vi "Init with SQL Record.vi"(8 "error in (no error)":errorcluster, 10 "MySQL Record":variant[](array[variant]), 11 "Banking Transaction in":refnum<class "Banking Transaction.lvclass">) -> (0 "error out":errorcluster, 3 "Banking Transaction out":refnum<class "Banking Transaction.lvclass">)   [LabVIEW 2018, in "Banking Transaction.lvclass"]
uses:
  Banking Transaction.lvclass
  Transaction/Transaction.lvclass
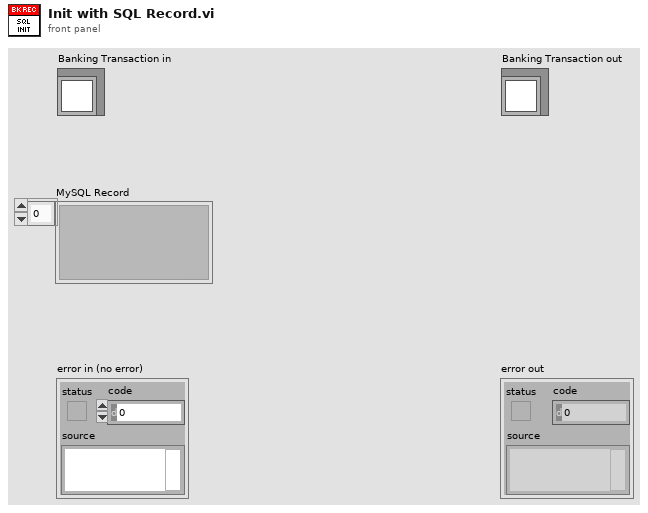
[diagram p1: front panel]
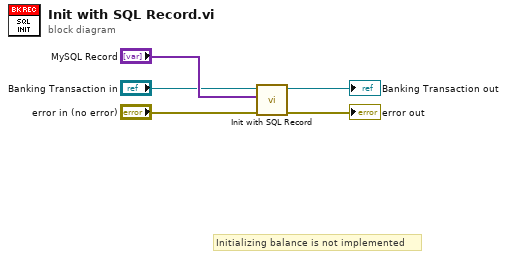
[diagram p0: block diagram]
diagram:
  # "Initializing balance is not implemented"
  n1 = call-parent "Init with SQL Record.vi"("error in (no error)"="error in (no error)", "MySQL Record"="MySQL Record", "Transaction in"="Banking Transaction in") -> ("error out"=→"error out":errorcluster, "Transaction out"=→"Banking Transaction out":refnum<class "Banking Transaction.lvclass">)  [unwired: 7 in]
